vi "TESTE ecart.vi"() -> ()   [LabVIEW 2026]
uses:
  <vilib>/numeric/Random Number (Range) DBL.vi
  <vilib>/ptbypt/NI_PtbyPt.lvlib
panel:
  in  "x":dbl=-1.0 format="%#_13g"
  in  "dephasage":bool
  in  "Choix Tension Y":T1(ring)=enum."10V"
  out "Graphe Y":cluster{"number":dbl, dbl}(graph)={"number"=43.75869499188818, 50.0}
  in  "frequency sin Y":dbl=2.0 caption="fréquence Y" format="%0.2f"
  in  "delta sin Y":dbl=1000.0
  out "dt sin Y":dbl
  in  "stop":bool
  in  "piezo start":bool
  in  "Model":T2(ring)=enum."sinus"
  in  "Choix Tension X":T1(ring)=enum."10V"
  out "Graphe X":cluster{"number":dbl, dbl}(graph)={"number"=10.0, 50.0}
  in  "frequency sin X":dbl=2.0 caption="fréquence" format="%0.2f"
  in  "delta sin X":dbl=1000.0
  out "dt sin X":dbl=7.597
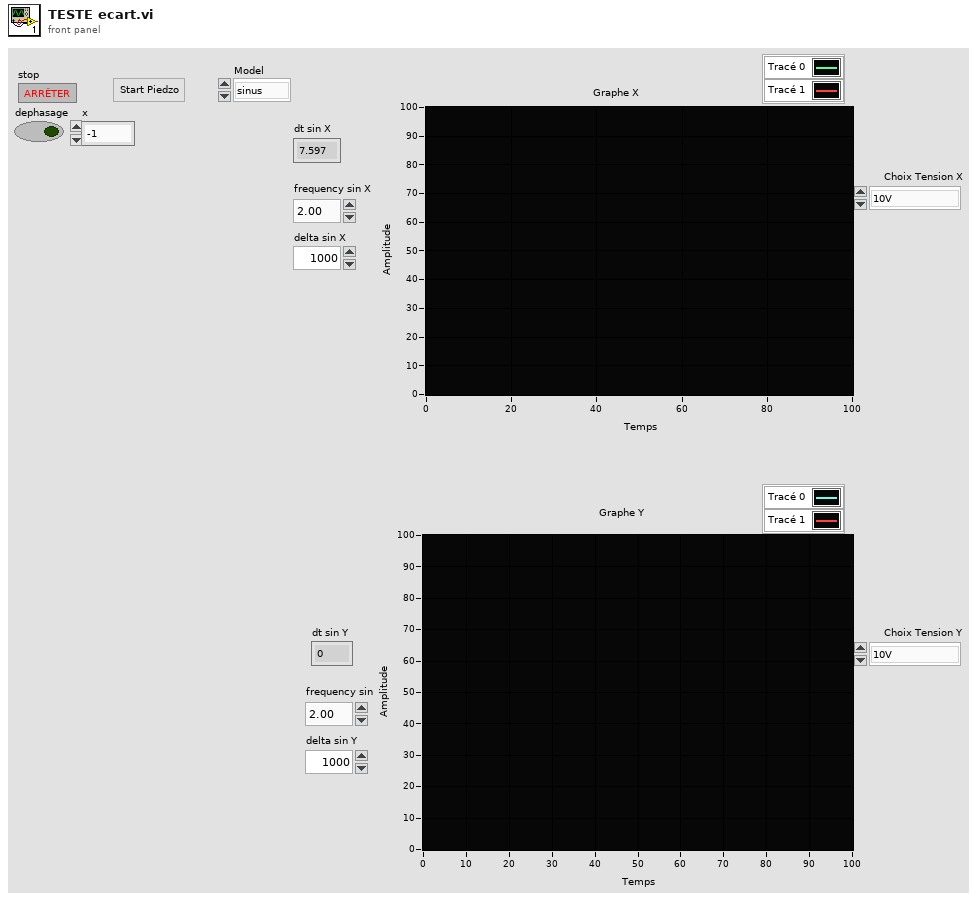
[diagram p1: front panel]
types:
  T1 = enum16{"0V", "10V", "20V", "30V", "40V", "50V", "60V", "70V", "80V", "90V", "100V"}
  T2 = enum16{"initial", "aléatoire", "gaussien", "sinus"}
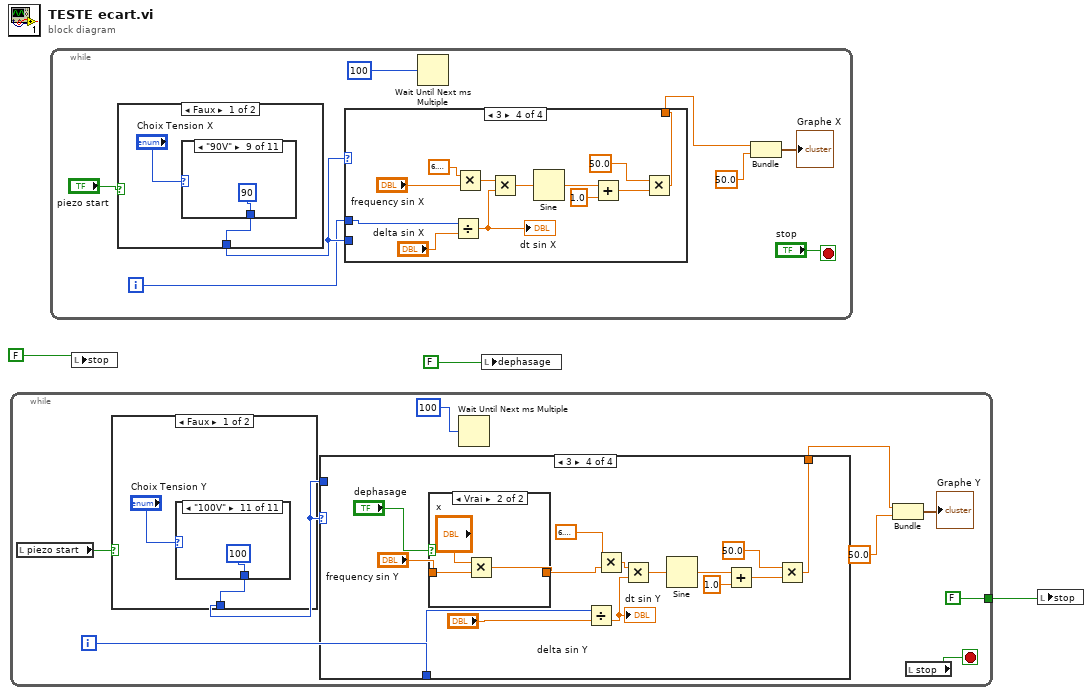
[diagram p0: block diagram]
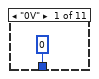
[diagram p2: hidden frame]
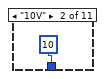
[diagram p3: hidden frame]
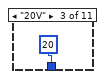
[diagram p4: hidden frame]
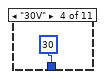
[diagram p5: hidden frame]
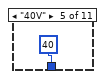
[diagram p6: hidden frame]
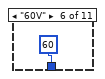
[diagram p7: hidden frame]
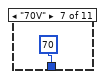
[diagram p8: hidden frame]
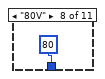
[diagram p9: hidden frame]
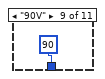
[diagram p10: hidden frame]
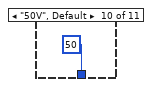
[diagram p11: hidden frame]
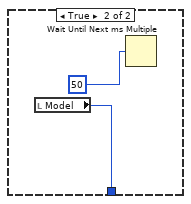
[diagram p12: hidden frame]
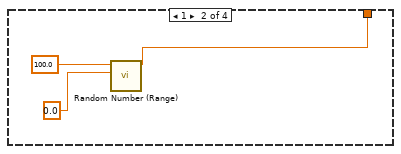
[diagram p14: hidden frame]
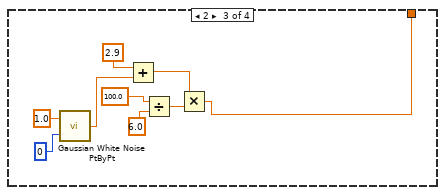
[diagram p15: hidden frame]
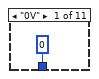
[diagram p17: hidden frame]
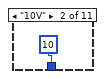
[diagram p18: hidden frame]
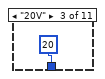
[diagram p19: hidden frame]
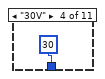
[diagram p20: hidden frame]
diagram:
  n1 = while {
    tunnel: [FALSE ("stop")] -> w2
    i -> [w8]
    stop <- w9 stop-if-true
    n2 = local read "piezo start"() -> (w6:bool)
    n3 = case shown="Faux" w6 {
      tunnel: [w14 w27] -> w10
      frame False {
        n4 = case shown="\"100V\"" "Choix Tension Y" {
          tunnel: [0 10 20 30 40 60 70 80 90 50 100] -> w14
          frame "0V" {
          }
          frame "10V" {
          }
          frame "20V" {
          }
          frame "30V" {
          }
          frame "40V" {
          }
          frame "60V" {
          }
          frame "70V" {
          }
          frame "80V" {
          }
          frame "90V" {
          }
          frame "50V", Default {
          }
          frame "100V" {
          }
        }
      }
      frame True {
        n5 = local read "Model"() -> (w27:T2)
        n6 = Wait Until Next ms Multiple(millisecond multiple=u32 50 ("n millisecondes")) -> ()  [unwired: 1 out]
      }
    }
    n7 = case shown="3" w10 {
      tunnel: [w28 w31 w32 w44] -> w5
      tunnel: w8 -> [_ _ _ w45]
      tunnel: w10 -> [w28 _ _ _]
      frame 0, Default {
      }
      frame 1 {
        n8 = call-poly <vilib>:"Random Number (Range).vi"("lower bound (0)"=0.0, "upper bound (100)"=100.0) -> ("number"=w31:dbl)  [unwired: 9 in]
      }
      frame 2 {
        n9 = call <vilib>:"Gaussian White Noise PtByPt.vi"("seed"=0, "standard deviation"=1.0) -> ("Gaussian white noise"=w38:dbl)  [unwired: 1 in]
        n10 = Add(x=2.9, y=w38) -> (x+y=w37:dbl)
        n11 = Divide(x=100.0, y=6.0) -> (x/y=w35:dbl)
        n12 = Multiply(x=w37, y=w35) -> (x*y=w32:dbl)
      }
      frame 3 {
        n13 = case shown="Vrai" "dephasage" {
          tunnel: "frequency sin Y" -> [w55 w58]
          tunnel: [w55 w57] -> w42
          frame False {
          }
          frame True {
            n14 = Multiply(x="x", y=w58) -> (x*y=w57:dbl)
          }
        }
        n15 = Divide(x=w45, y="delta sin Y") -> (x/y=w48:dbl)
        "dt sin Y" <- w48
        n16 = Multiply(x=6.283185307179586, y=w42) -> (x*y=w46:dbl)
        n17 = Multiply(x=w46, y=w48) -> (x*y=w49:dbl)
        n18 = Sine(x=w49) -> (sin(x)=w50:dbl)
        n19 = Add(x=w50, y=1.0) -> (x+y=w51:dbl)
        n20 = Multiply(x=50.0, y=w51) -> (x*y=w44:dbl)
      }
    }
    n21 = Wait Until Next ms Multiple(millisecond multiple=u32 100 ("time Y")) -> ()  [unwired: 1 out]
    n22 = Bundle("number"=w5, 50.0) -> (→"Graphe Y":cluster{"number":dbl, dbl})  [unwired: 1 in]
    n23 = local read "stop"() -> (w9:bool)
  }
  n24 = while {
    i -> [w60]
    stop <- "stop" stop-if-true
    n25 = case shown="Faux" "piezo start" {
      tunnel: [w68 "Model"] -> w66
      frame False {
        n26 = case shown="\"90V\"" "Choix Tension X" {
          tunnel: [0 10 20 30 40 60 70 80 90 50 100] -> w68
          frame "0V" {
          }
          frame "10V" {
          }
          frame "20V" {
          }
          frame "30V" {
          }
          frame "40V" {
          }
          frame "60V" {
          }
          frame "70V" {
          }
          frame "80V" {
          }
          frame "90V" {
          }
          frame "50V", Default {
          }
          frame "100V" {
          }
        }
      }
      frame True {
      }
    }
    n27 = case shown="3" w66 {
      tunnel: [w81 w83 w85 w94] -> w64
      tunnel: w60 -> [_ _ _ w95]
      tunnel: w66 -> [w81 _ _ _]
      frame 0, Default {
      }
      frame 1 {
        n28 = call-poly <vilib>:"Random Number (Range).vi"("lower bound (0)"=0.0, "upper bound (100)"=100.0) -> ("number"=w83:dbl)  [unwired: 9 in]
      }
      frame 2 {
        n29 = call <vilib>:"Gaussian White Noise PtByPt.vi"("seed"=0, "standard deviation"=1.0) -> ("Gaussian white noise"=w91:dbl)  [unwired: 1 in]
        n30 = Add(x=3.0, y=w91) -> (x+y=w90:dbl)
        n31 = Divide(x=100.0, y=6.0) -> (x/y=w88:dbl)
        n32 = Multiply(x=w90, y=w88) -> (x*y=w85:dbl)
      }
      frame 3 {
        n33 = Divide(x=w95, y="delta sin X") -> (x/y=w102:dbl)
        "dt sin X" <- w102
        n34 = Multiply(x=6.283185307179586, y="frequency sin X") -> (x*y=w104:dbl)
        n35 = Multiply(x=w104, y=w102) -> (x*y=w101:dbl)
        n36 = Sine(x=w101) -> (sin(x)=w100:dbl)
        n37 = Add(x=w100, y=1.0) -> (x+y=w99:dbl)
        n38 = Multiply(x=50.0, y=w99) -> (x*y=w94:dbl)
      }
    }
    n39 = Wait Until Next ms Multiple(millisecond multiple=u32 100 ("n millisecondes")) -> ()  [unwired: 1 out]
    n40 = Bundle("number"=w64, 50.0) -> (→"Graphe X":cluster{"number":dbl, dbl})  [unwired: 1 in]
  }
  n41 = local write "stop"(FALSE ("stop")) -> ()
  n42 = local write "dephasage"(FALSE) -> ()
  n43 = local write "stop"(w2) -> ()
